vi "Is Valid Number (SGL Array).vi"(2 "SGL Array":sgl[](array[numeric])) -> (7 "Is Valid Number? (1D)":bool[](array[boolean]))   [LabVIEW 2021, in "Comparison.lvlib"]
uses:
  Comparison.lvlib
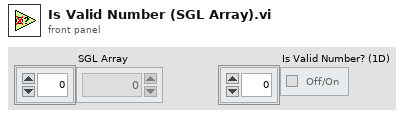
[diagram p1: front panel]
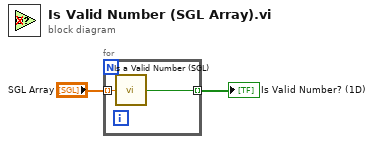
[diagram p0: block diagram]
diagram:
  n1 = for {
    tunnel: "SGL Array" -> [w4] mode=indexing
    tunnel: [w3] -> w2 mode=indexing
    n2 = call "Is a Valid Number (SGL).vi"("Number"=w4) -> ("Valid Number?"=w3:bool)  [unwired: 8 in]
  }
  "Is Valid Number? (1D)" <- w2
